vi "Add Sensor.vi"(0 "Sensors in":T1[](array[typedef]) {"Max Error % of Reading" format="%.2f"; "Max Stability Error" format="%.2f"; "Max Mean Squared Error" format="%.2f"; "Max Error % of Full Scale" format="%.2f"; "Coefficients" format="%.2f"; "Voltage List" format="%.2f"; "EGU List" format="%.2f"; "EGU Range"."Low Limit" format="%.2f"; "EGU Range"."High Limit" format="%.2f"; "Voltage Range"."Low Limit" format="%.2f"; "Voltage Range"."High Limit" format="%.2f"; "Last Cal Info"."Last Calibration Date" format="%.2f"}, 5 "Sensor Name in":string) -> (4 "Sensors out":T1[](array[typedef]) {"Max Error % of Reading" format="%.2f"; "Max Stability Error" format="%.2f"; "Max Mean Squared Error" format="%.2f"; "Max Error % of Full Scale" format="%.2f"; "Coefficients" format="%.2f"; "Voltage List" format="%.2f"; "EGU List" format="%.2f"; "EGU Range"."Low Limit" format="%.2f"; "EGU Range"."High Limit" format="%.2f"; "Voltage Range"."Low Limit" format="%.2f"; "Voltage Range"."High Limit" format="%.2f"; "Last Cal Info"."Last Calibration Date" format="%.2f"}, 6 "Sensor Name out":string)   [LabVIEW 2023]
uses:
  Type Defs and Controls/Sensor.ctl
  <vilib>/Analysis/NI_AALPro.lvlib
panel:
  in  "Units":bool
  out "Units":string
  in  "Cancel":bool
  in  "OK":bool
  in  "EGU Range":cluster{"EGU High":dbl, "EGU Low":dbl}
  in  "Voltage Range":cluster{"Voltage High":dbl, "Voltage Low":dbl}
  in  "Sensor Name":string
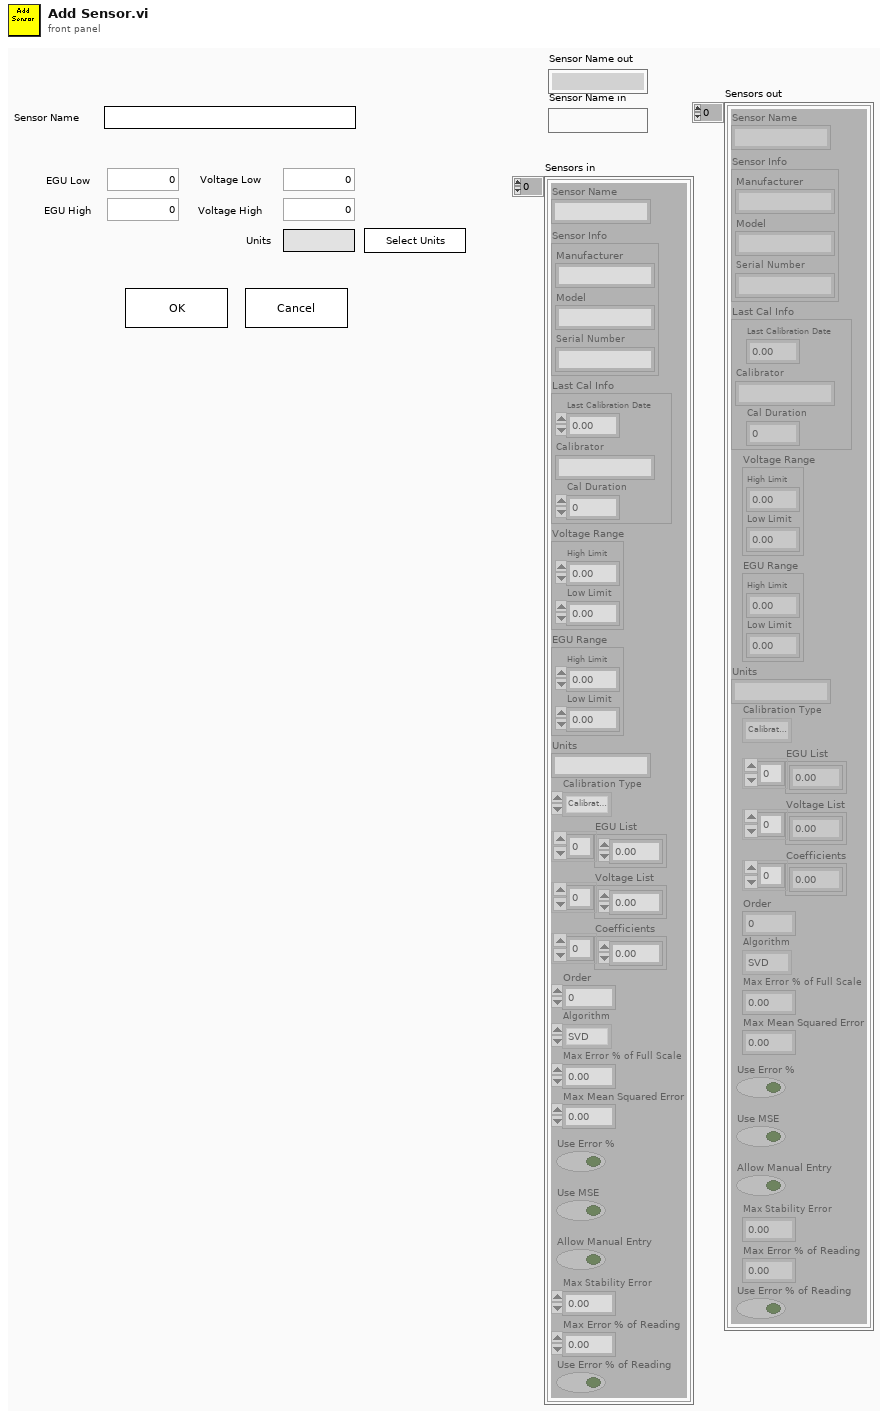
[diagram p1: front panel]
types:
  T1 = typedef "Sensor.ctl" = cluster{"Sensor Name":string, "Sensor Info":cluster{"Manufacturer":string, "Model":string, "Serial Number":string}, "Last Cal Info":cluster{"Last Calibration Date":dbl, "Calibrator":string, "Cal Duration":i32}, "Voltage Range":cluster{"High Limit":dbl, "Low Limit":dbl}, "EGU Range":cluster{"High Limit":dbl, "Low Limit":dbl}, "Units":string, "Calibration Type":enum16{"Calibrate Analog", "Compare Analog Calibration"}, "EGU List":dbl[], "Voltage List":dbl[], "Coefficients":dbl[], "Order":i32, "Algorithm":enum32{"SVD", "Givens", "Givens2", "Householder", "LU Decomposition", "Cholesky"}, "Max Error % of Full Scale":dbl, "Max Mean Squared Error":dbl, "Use Error %":bool, "Use MSE":bool, "Allow Manual Entry":bool, "Max Stability Error":dbl, "Max Error % of Reading":dbl, "Use Error % of Reading":bool}
  T2 = cluster{"Last Calibration Date":dbl, "Calibrator":string, "Cal Duration":i32}
  T3 = enum16{"Calibrate Analog", "Compare Analog Calibration"}
  T4 = enum32{"SVD", "Givens", "Givens2", "Householder", "LU Decomposition", "Cholesky"}
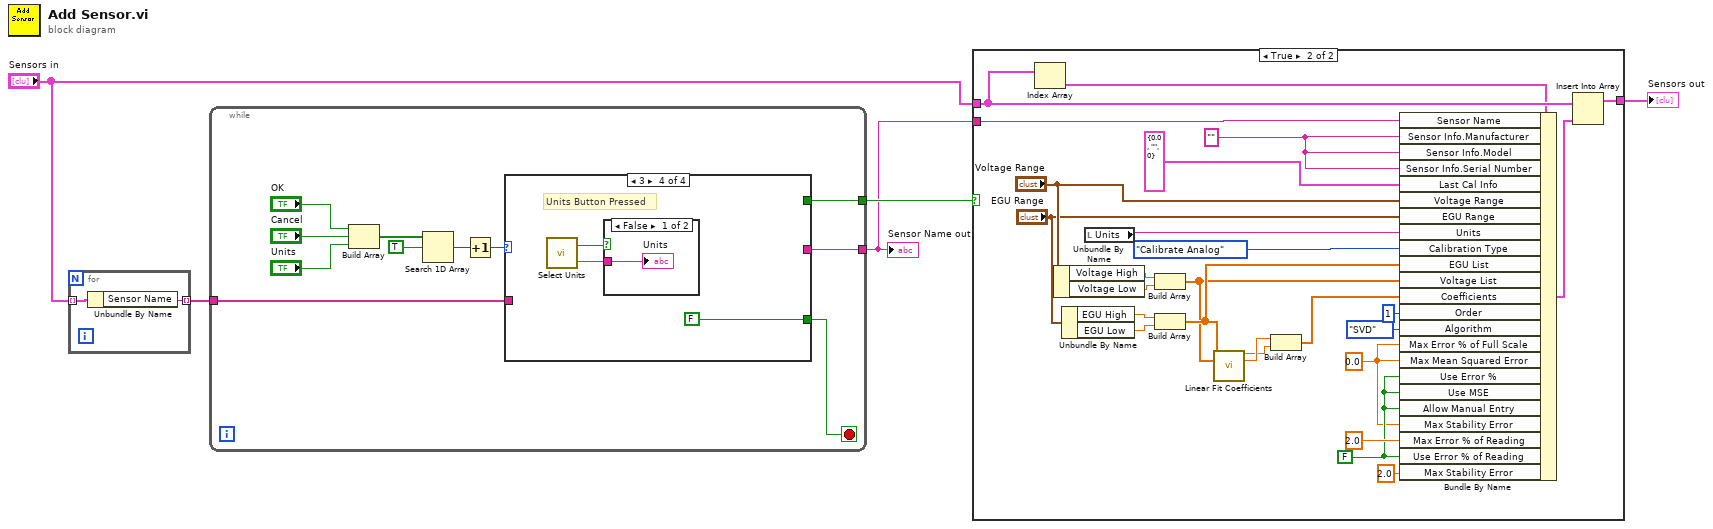
[diagram p0: block diagram]
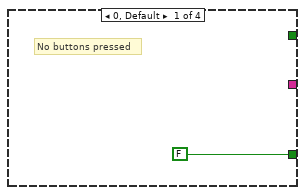
[diagram p3: hidden frame]
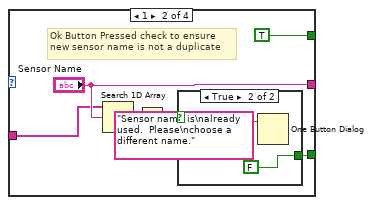
[diagram p4: hidden frame]
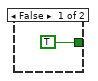
[diagram p5: hidden frame]
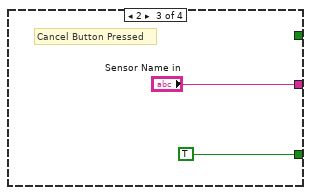
[diagram p6: hidden frame]
diagram:
  n1 = for {
    tunnel: "Sensors in" -> [w7] mode=indexing
    tunnel: [w6] -> w1 mode=indexing
    n2 = Unbundle By Name(w7) -> ("Sensor Name"=w6:string)
  }
  n3 = while {
    tunnel: [w11] -> w3
    tunnel: [w9] -> w5
    tunnel: w1 -> [w8]
    stop <- w10 stop-if-true
    n4 = Build Array("OK", "Cancel", "Units") -> (w15:bool[])
    n5 = Search 1D Array(1D array=w15, element=TRUE) -> (index of element=w13:i32)  [unwired: 1 in]
    n6 = Increment(x=w13) -> (x+1=w12:i32)
    n7 = case shown="3" w12 {
      tunnel: [FALSE w20 TRUE FALSE] -> w10
      tunnel: [_ "Sensor Name" "Sensor Name in" _] -> w11
      tunnel: [_ TRUE _ _] -> w9
      tunnel: w8 -> [_ w23 _ _]
      frame 0, Default {
        # "No buttons pressed"
      }
      frame 1 {
        # "Ok Button Pressed check to ensure\nnew sensor name is not a duplicate"
        n8 = Search 1D Array(1D array=w23, element="Sensor Name") -> (index of element=w22:i32)  [unwired: 1 in]
        n9 = Greater Or Equal To 0?(x=w22) -> (x >= 0?=w21:bool)
        n10 = case shown="True" w21 {
          tunnel: [TRUE FALSE] -> w20
          frame False {
          }
          frame True {
            n11 = One Button Dialog(message="Sensor name is\nalready used.  Please\nchoose a different name.") -> ()  [unwired: 1 in, 1 out]
          }
        }
      }
      frame 2 {
        # "Cancel Button Pressed"
      }
      frame 3 {
        # "Units Button Pressed"
        n12 = call "Select Units.vi"() -> ("Element"=w33:string, "Cancelled"=w32:bool)  [unwired: 4 in]
        n13 = case shown="False" w32 {
          tunnel: w33 -> [w34 _]
          frame False {
            "Units" <- w34
          }
          frame True {
          }
        }
      }
    }
  }
  "Sensor Name out" <- w3
  n14 = case shown="True" w5 {
    tunnel: "Sensors in" -> [w35 w61]
    tunnel: [w35 w58] -> w4
    tunnel: w3 -> [_ w52]
    frame False {
    }
    frame True {
      w51 = "" ("Sensor Info.Manufacturer")
      w48 = 0.0 ("Max Stability Error")
      w49 = FALSE ("Use Error % of Reading")
      n15 = Index Array(array=w61) -> (element=w60:T1)  [unwired: 1 in]
      n16 = Unbundle By Name("Voltage Range") -> ("Voltage High"=w45:dbl, "Voltage Low"=w44:dbl)
      n17 = Unbundle By Name("EGU Range") -> ("EGU High"=w43:dbl, "EGU Low"=w42:dbl)
      n18 = local read "Units"() -> (w53:string)
      n19 = Build Array(w45, w44) -> (w40:dbl[])
      n20 = Build Array(w43, w42) -> (w41:dbl[])
      n21 = call <vilib>:"Linear Fit Coefficients.vi"("Y"=w41, "X"=w40) -> ("slope"=w36:dbl, "intercept"=w37:dbl)  [unwired: 11 in, 1 out]
      n22 = Build Array(w37, w36) -> (w39:dbl[])
      n23 = Bundle By Name(cluster=w60, "Sensor Name"=w52, "Sensor Info.Manufacturer"=w51, "Sensor Info.Model"=w51, "Sensor Info.Serial Number"=w51, "Last Cal Info"=T2 {"Last Calibration Date"=0.0, "Calibrator"="", "Cal Duration"=0}, "Voltage Range"="Voltage Range", "EGU Range"="EGU Range", "Units"=w53, "Calibration Type"=T3."Calibrate Analog", "EGU List"=w41, "Voltage List"=w40, "Coefficients"=w39, "Order"=1, "Algorithm"=T4."SVD", "Max Error % of Full Scale"=w48, "Max Mean Squared Error"=w48, "Use Error %"=w49, "Use MSE"=w49, "Allow Manual Entry"=w49, "Max Stability Error"=w48, "Max Error % of Reading"=2.0, "Use Error % of Reading"=w49, "Max Stability Error"=2.0) -> (w59:T1)
      n24 = Insert Into Array(array=w61, new element=w59) -> (w58:T1[])  [unwired: 1 in]
    }
  }
  "Sensors out" <- w4
